vi "Main Menu.vi"() -> ()   [LabVIEW 2020]
panel:
  in  "Find Segment":bool
  in  "Analyze Button":bool
  in  "Step Size (seconds)":dbl=0.01 min=0.01 max=1.0 step=0.05
  in  "Window Size (seconds)":dbl=0.01 min=0.01 max=1.0 step=0.05
  in  "Segment Button":bool
  in  "Open Button":bool
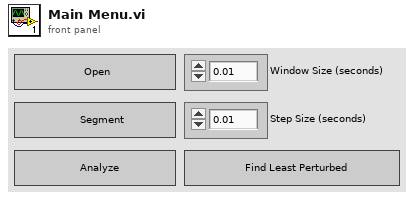
[diagram p1: front panel]
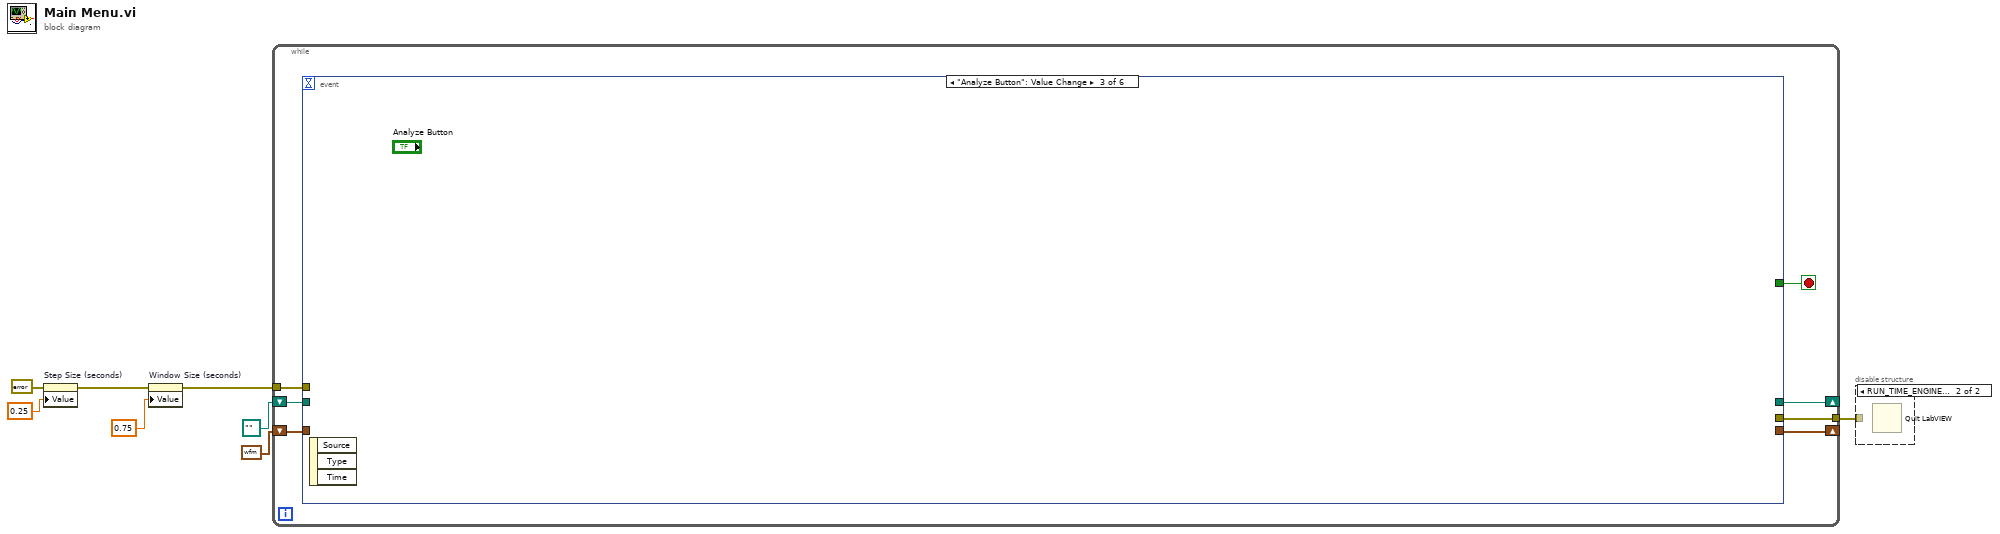
[diagram p0: block diagram]
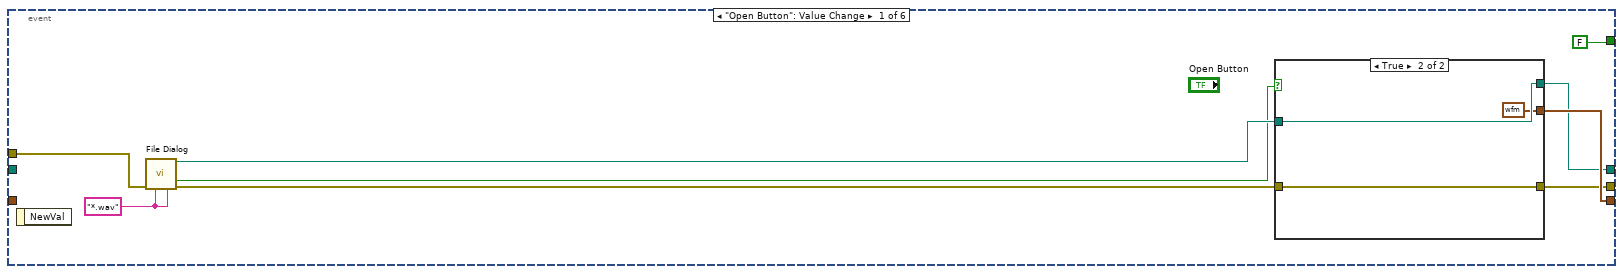
[diagram p3: hidden frame]
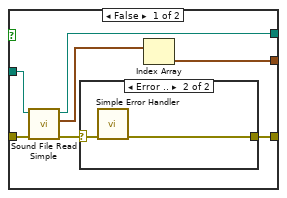
[diagram p4: hidden frame]
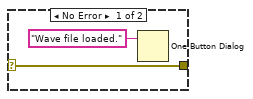
[diagram p5: hidden frame]
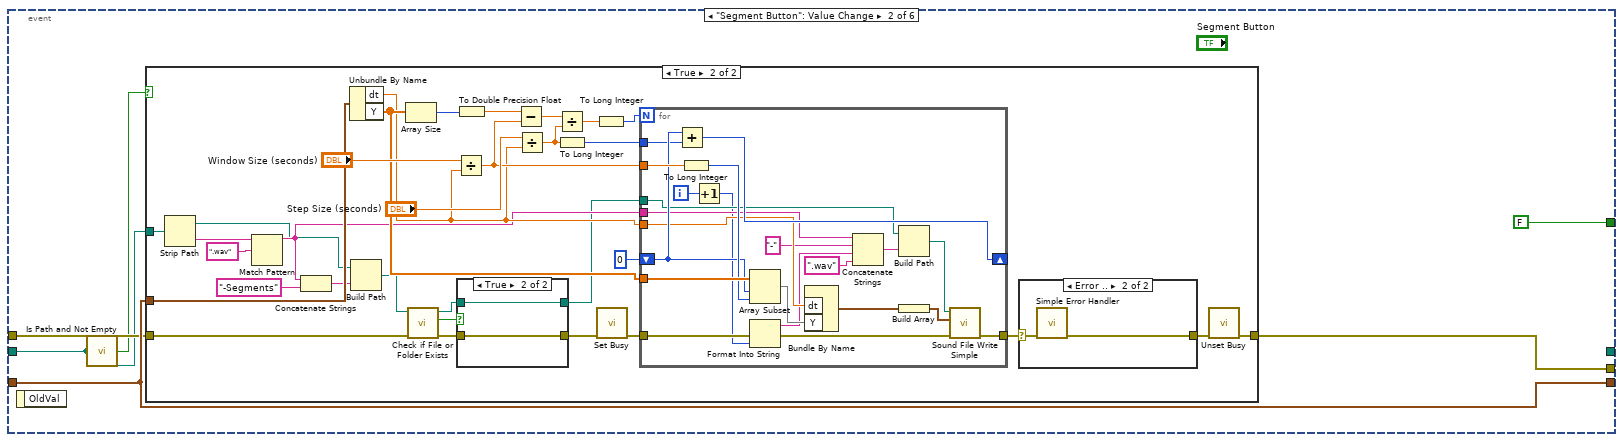
[diagram p6: hidden frame]
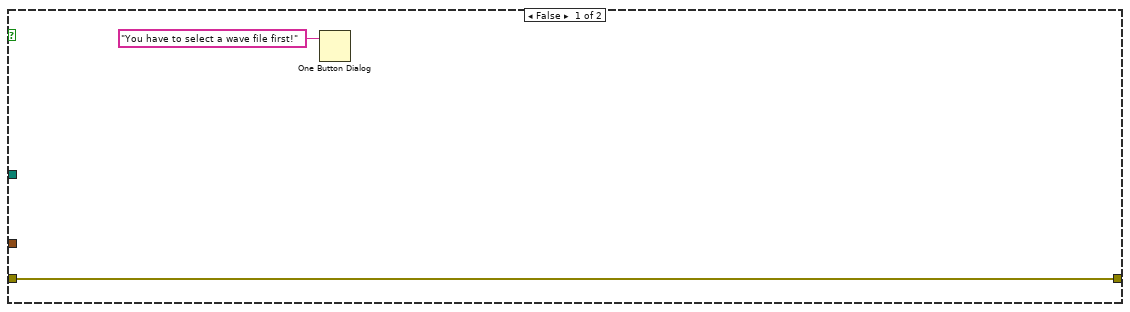
[diagram p7: hidden frame]
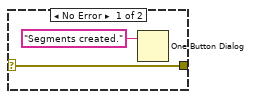
[diagram p8: hidden frame]
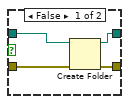
[diagram p9: hidden frame]
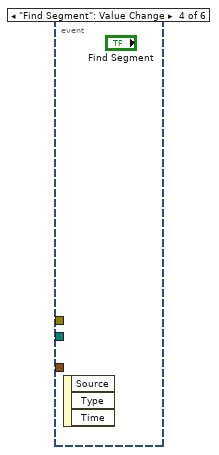
[diagram p10: hidden frame]
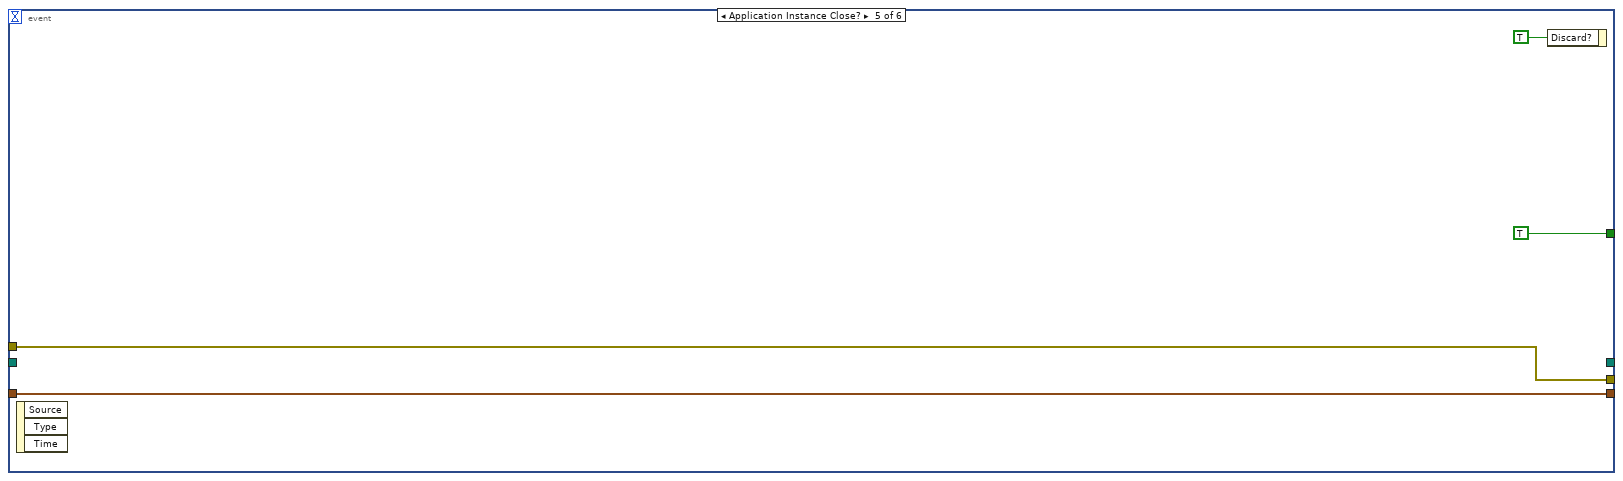
[diagram p11: hidden frame]
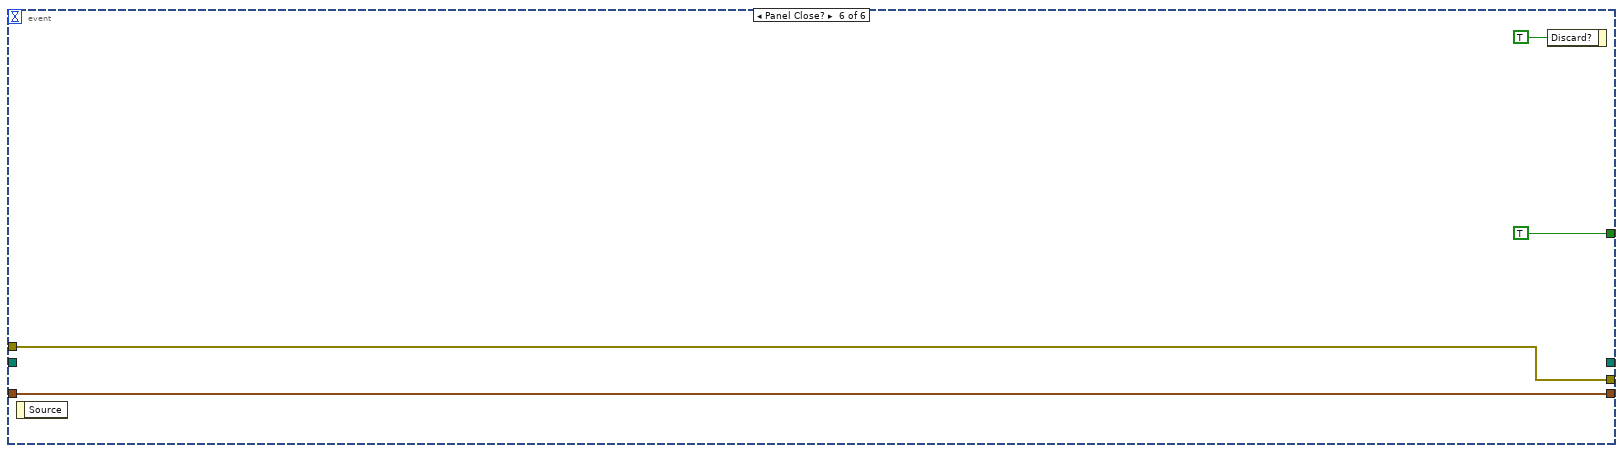
[diagram p12: hidden frame]
diagram:
  n1 = property on="Step Size (seconds)" class="DigNum (strict)"(error in=errorcluster {"status"=FALSE, "code"=0, "source"=""} ("error in (no error)"), "Value"=0.25 ("Step Size (seconds)")) -> (error out=w4:errorcluster)  [unwired: 1 in, 1 out]
  n2 = property on="Window Size (seconds)" class="DigNum (strict)"(error in=w4, "Value"=0.75 ("Window Size (seconds)")) -> (error out=w3:errorcluster)  [unwired: 1 in, 1 out]
  n3 = while {
    shift-right: [w14] -> _
    shift-left: waveform(dbl) {"t0"=timestamp(0 s since 1904-01-01), "dt"=1.0, "Y"=[]} ("element") -> [w13]
    shift-right: [w12] -> _
    shift-left: path "" ("path out") -> [w11]
    tunnel: w3 -> [w10]
    tunnel: [w9] -> w1
    stop <- w15 stop-if-true
    n4 = event shown="[2] \"Analyze Button\": Value Change" {
      selector: _ -> [_ _ _ _ _ _]
      dyn-events: _ -> [_ _ _ _ _ _]
      timeout: _ -> [_ _ _ _ _ _]
      tunnel: [FALSE FALSE _ _ TRUE TRUE] -> w15
      tunnel: [w21 w43 _ _ w113 w116] -> w14
      tunnel: w13 -> [_ w43 _ _ w113 w116]
      tunnel: [w20 _ _ _ _ _] -> w12
      tunnel: w11 -> [_ w40 _ _ _ _]
      tunnel: w10 -> [w19 w41 _ _ w111 w115]
      tunnel: [w18 w42 _ _ w111 w115] -> w9
      event "Open Button": Value Change {
        w24 = "*.wav" ("pattern label")
        n5 = event-data() -> ()  [unwired: 1 in, 1 out]
        n6 = call "File Dialog"("error in"=w19, "pattern (all files)"=w24, "pattern label"=w24) -> ("selected path"=w22:path, "cancelled"=w16:bool, "error out"=w23:errorcluster)  [unwired: 9 in, 1 out]
        n7 = case shown="True" w16 {
          tunnel: w23 -> [w31 w37]
          tunnel: w22 -> [w30 w38]
          tunnel: [w28 waveform(dbl) {"t0"=timestamp(0 s since 1904-01-01), "dt"=1.0, "Y"=[]} ("data")] -> w21
          tunnel: [w27 w38] -> w20
          tunnel: [w25 w37] -> w18
          frame False {
            n8 = call <vilib>:"Sound File Read Simple.vi"("error in (no error)"=w31, "path"=w30) -> ("error out"=w26:errorcluster, "data"=w29:waveform(dbl)[], "path out"=w27:path)  [unwired: 6 in, 1 out]
            n9 = case shown="Error .." w26 {
              selector: w26 -> [w33 w35]
              tunnel: [w33 w34] -> w25
              frame No Error {
                n10 = One Button Dialog(message="Wave file loaded.") -> ()  [unwired: 1 in, 1 out]
              }
              frame Error {
                n11 = call <vilib>:"Simple Error Handler.vi"("error in (no error)"=w35) -> ("error out"=w34:errorcluster)  [unwired: 4 in, 4 out]
              }
            }
            n12 = Index Array(array=w29) -> (element=w28:waveform(dbl))  [unwired: 1 in]
          }
          frame True {
          }
        }
      }
      event "Segment Button": Value Change {
        n13 = event-data() -> ()  [unwired: 1 in, 1 out]
        n14 = call <vilib>:"Is Path and Not Empty.vi"("path"=w40) -> ("Is Path and Not Empty?"=w39:bool)  [unwired: 4 in]
        n15 = case shown="True" w39 {
          tunnel: w43 -> [_ w66]
          tunnel: [w46 w64] -> w42
          tunnel: w41 -> [w46 w59]
          tunnel: w40 -> [_ w47]
          frame False {
            n16 = One Button Dialog(message="You have to select a wave file first!") -> ()  [unwired: 1 in, 1 out]
          }
          frame True {
            n17 = Strip Path(path=w47) -> (stripped path=w49:path, name=w61:string)
            n18 = Match Pattern(string=w61, regular expression=".wav") -> (before substring=w60:string)  [unwired: 1 in, 3 out]
            n19 = Concatenate Strings(w60, "-Segments" ("string")) -> (w50:string)
            n20 = Unbundle By Name(w66) -> ("dt"=w67:dbl, "Y"=w71:dbl[])
            n21 = Build Path(base path=w49, name or relative path=w50) -> (appended path=w51:path)
            n22 = Array Size(array=w71) -> (size(s)=w76:i32)
            n23 = call <vilib>:"Check if File or Folder Exists.vi"("error in (no error)"=w59, "path"=w51) -> ("error out"=w56:errorcluster, "file or folder exists?"=w57:bool, "dup path"=w54:path)  [unwired: 7 in]
            n24 = Divide(x="Window Size (seconds)", y=w67) -> (x/y=w70:dbl)
            n25 = To Double Precision Float(number=w76) -> (double precision float=w75:dbl)
            n26 = case shown="True" w57 {
              tunnel: w56 -> [w86 w88]
              tunnel: [w85 w88] -> w55
              tunnel: w54 -> [w84 w87]
              tunnel: [w83 w87] -> w48
              frame False {
                n27 = Create Folder(path (use dialog)=w84, error in=w86) -> (created path=w83:path, error out=w85:errorcluster)  [unwired: 1 in, 1 out]
              }
              frame True {
              }
            }
            n28 = Subtract(x=w75, y=w70) -> (x-y=w74:dbl)
            n29 = Divide(x="Step Size (seconds)", y=w67) -> (x/y=w68:dbl)
            n30 = Divide(x=w74, y=w68) -> (x/y=w72:dbl)
            n31 = To Long Integer(number=w68) -> (32bit integer=w63:i32)
            n32 = To Long Integer(number=w72) -> (32bit integer=w73:i32)
            n33 = call <vilib>:"Set Busy.vi"("error in (no error)"=w55) -> ("error out"=w65:errorcluster)  [unwired: 9 in, 1 out]
            n34 = for {
              N: w73 -> [_]
              tunnel: w71 -> [w110]
              tunnel: w70 -> [w108]
              shift-right: [w106] -> _
              shift-left: 0 -> [w107]
              tunnel: w67 -> [w104]
              tunnel: w65 -> [w97]
              tunnel: [w95] -> w53
              tunnel: w63 -> [w94]
              tunnel: w48 -> [w93]
              tunnel: w60 -> [w92]
              i -> [w90]
              n35 = Add(x=w107, y=w94) -> (x+y=w106:i32)
              n36 = To Long Integer(number=w108) -> (32bit integer=w109:i32)
              n37 = Increment(x=w90) -> (x+1=w89:i32)
              n38 = Array Subset(array=w110, index=w107, length=w109) -> (w105:dbl[])
              n39 = Format Into String(error in=w97, w89) -> (resulting string=w100:string, error out=w96:errorcluster)  [unwired: 2 in]
              n40 = Bundle By Name("dt"=w104, "Y"=w105) -> (w102:waveform(dbl))  [unwired: 1 in]
              n41 = Concatenate Strings(w92, "-" ("string"), w100, ".wav" ("regular expression")) -> (w99:string)
              n42 = Build Path(base path=w93, name or relative path=w99) -> (appended path=w98:path)
              n43 = Build Array(w102) -> (w103:waveform(dbl)[])
              n44 = call <vilib>:"Sound File Write Simple.vi"("error in (no error)"=w96, "data"=w103, "path"=w98) -> ("error out"=w95:errorcluster)  [unwired: 7 in, 1 out]
            }
            n45 = case shown="Error .." w53 {
              selector: w53 -> [w80 w82]
              tunnel: [w80 w81] -> w52
              frame No Error {
                n46 = One Button Dialog(message="Segments created.") -> ()  [unwired: 1 in, 1 out]
              }
              frame Error {
                n47 = call <vilib>:"Simple Error Handler.vi"("error in (no error)"=w82) -> ("error out"=w81:errorcluster)  [unwired: 4 in, 4 out]
              }
            }
            n48 = call <vilib>:"Unset Busy.vi"("error in (no error)"=w52) -> ("error out"=w64:errorcluster)  [unwired: 10 in]
          }
        }
      }
      event "Analyze Button": Value Change {
        n49 = event-data() -> ()  [unwired: 1 in, 3 out]
      }
      event "Find Segment": Value Change {
        n50 = event-data() -> ()  [unwired: 1 in, 3 out]
      }
      event Application Instance Close? {
        n51 = event-data() -> ()  [unwired: 1 in, 3 out]
        n52 = event-data("Discard?"=TRUE) -> ()  [unwired: 1 in, 1 out]
      }
      event Panel Close? {
        n53 = event-data() -> ()  [unwired: 1 in, 1 out]
        n54 = event-data("Discard?"=TRUE) -> ()  [unwired: 1 in, 1 out]
      }
    }
  }
  n55 = disable-structure shown="RUN_TIME_ENGINE==True" {
    disable-tunnel: w1 -> [_ _]
    frame condition #0 (active) {
    }
    frame condition #1 {
      n56 = Quit LabVIEW() -> ()  [unwired: 1 in]
    }
  }
